vi "Tarea 8.vi"() -> ()   [LabVIEW 2020]
uses:
  <vilib>/addons/Control Design/_Model Construction/Model Creation.llb/Model Creation SubVI/cd_Create State Space Model.vi
  <vilib>/addons/Control Design/_Time Response Analysis/Time Response.llb/Time Response subVI/cd_Step Response (State-Space).vi
  <vilib>/addons/Control Design/_Dynamic Analysis/Dynamic Analysis.llb/Dynamic Analysis subVI/cd_Root Locus (State-Space).vi
  <vilib>/addons/Control Design/_Dynamic Analysis/Dynamic Analysis.llb/Dynamic Analysis subVI/cd_Poles (State-Space).vi
  <vilib>/addons/Control Design/_Utility/Model Viewer.llb/Model Viewer SubVI/cd_Draw Transfer Function Equation (SS).vi
  <vilib>/addons/Control Design/_Utility/Model Viewer.llb/Model Viewer SubVI/cd_Draw State-Space Equation (SS).vi
  <vilib>/imath/engines/lvmath/Plug In/Control Design/BuiltInFunctions/ackermann/NIMS_CD_ackermann(A,B,poles,STR).vi
  <vilib>/imath/engines/lvmath2/RunTimeEngine/ArithmeticOperatorToken/NIMS_ArithmeticOperator_multmx.vi
  <instcachedir>/0/NIMS_ArithmeticOperator_multmx_177F0753FB7A49B190E35F5DD0E80316.lvgen/NIMS_ArithmeticOperator_multmx_177F0753FB7A49B190E35F5DD0E80316_004.vi
  <vilib>/imath/engines/lvmath2/RunTimeEngine/ArithmeticOperatorToken/NIMS_ArithmeticOperator_minus.vi
  <instcachedir>/0/NIMS_ArithmeticOperator_minus_822089A08BE049DB927E6BEA78E100F1.lvgen/NIMS_ArithmeticOperator_minus_822089A08BE049DB927E6BEA78E100F1_002.vi
  <vilib>/imath/engines/lvmath2/RunTimeSupport/NIMS_Get Scalar_w Error.vi
  <instcachedir>/0/NIMS_Get Scalar_w Error_5A0E401CB6154DCF81784DB8E431B6E1.lvgen/NIMS_Get Scalar_w Error_5A0E401CB6154DCF81784DB8E431B6E1_003.vi
  <vilib>/imath/engines/lvmath2/RunTimeEngine/BuiltInFunctions/ss_to_tf/NIMS_ss_to_tf(4i).vi
  <vilib>/imath/engines/lvmath2/RunTimeEngine/ErrorHandling/NIMS_Create Error From Enums.vi
  <vilib>/imath/engines/lvmath/Plug In/Control Design/BuiltInFunctions/tf/NIMS_CD_tf(num,den,Ts).vi
  <vilib>/imath/engines/lvmath2/RunTimeEngine/NodeEndStatement/NIMS_NodeEndStatement_Output.vi
  <instcachedir>/0/NIMS_NodeEndStatement_Output_53EC0D466D134D7ABD903AC30B43404B.lvgen/NIMS_NodeEndStatement_Output_53EC0D466D134D7ABD903AC30B43404B_010.vi
  <instcachedir>/0/NIMS_NodeEndStatement_Output_53EC0D466D134D7ABD903AC30B43404B.lvgen/NIMS_NodeEndStatement_Output_53EC0D466D134D7ABD903AC30B43404B_005.vi
  <vilib>/imath/engines/lvmath2/RunTimeEngine/ErrorHandling/NIMS_Finalize Error.vi
  <vilib>/addons/Control Design/_Utility/Model Viewer.llb/Model Viewer SubVI/cd_Draw Transfer Function Equation (TF).vi
  <vilib>/addons/Control Design/_Utility/NI_CD_Model Viewer.lvlib
  <vilib>/addons/Control Design/_Model Construction/NI_LinSys_Model Creation.lvlib
  <vilib>/addons/Control Design/_State-Space Analysis/NI_CD_State-Space Analysis.lvlib
  <vilib>/addons/Control Design/_Dynamic Analysis/NI_CD_Dynamic Analysis.lvlib
  <vilib>/addons/Control Design/_Time Response Analysis/NI_CD_Time Response.lvlib
panel:
  out "TFO Equation":picture
  in  "Polos Observador":cdb[](array[numeric])=[-8.0+0.0i, -8.0+0.0i]
  out "ke":dbl[](array[numeric])
  out "Step Response Graph":cluster{"time":dbl[], dbl[]}[](graph)
  out "Root Locus Graph":cluster{dbl[], dbl[]}[](graph)
  out "Poles":cdb[](array[numeric]) format="%.3f"
  in  "Polos":cdb[](array[numeric])=[-2.0+3.4641i, -2.0-3.4641i, -10.0+0.0i]
  out "K":dbl[](array[numeric])
  out "Transfer Function Equation":picture
  out "Is Observable?":bool
  out "Observability  Matrix":dbl[][](array[numeric]) format="%#.2g"
  out "Is Controllable?":bool
  out "Controllability Matrix":dbl[][](array[numeric])=[[1.0, 0.0, 6.0], [0.0, 1.0, -1.0], [0.0, 0.0, 0.0]] format="%.2f"
  out "State Equation":picture
  in  "D":dbl[][](array[numeric])=[[1.0]]
  in  "C":dbl[][](array[numeric])=[[1.0, 1.0, 1.0]]
  in  "B":dbl[][](array[numeric])=[[1.0], [1.0], [1.0]]
  in  "A":dbl[][](array[numeric])=[[1.0, 1.0, 1.0], [1.0, 1.0, 1.0], [1.0, 1.0, 1.0]]
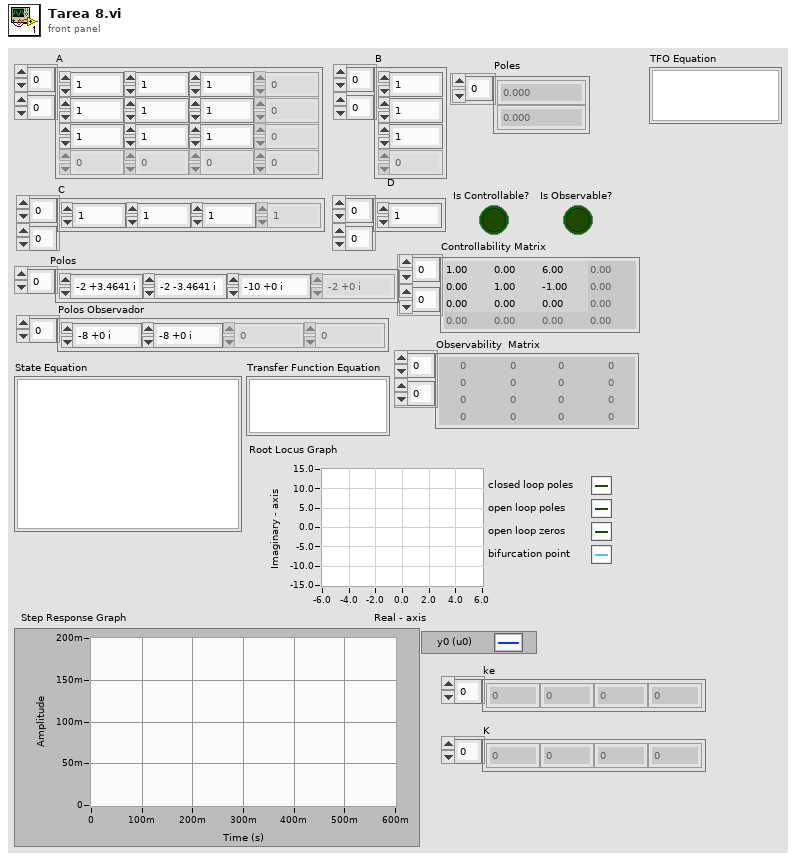
[diagram p1: front panel]
types:
  T1 = typedef "NI_LinSys_Model Typedefs.lvlib/CD State Space Model (MIMO).ctl" = cluster{"properties":T2, "A":dbl[][], "B":dbl[][], "C":dbl[][], "D":dbl[][], "StateNames":string[], "Transport Delay":dbl[][]}
  T2 = typedef "NI_LinSys_Model Typedefs.lvlib/CD General Elements.ctl" = cluster{"Model name":string, "Input names":string[], "Output names":string[], "Input Delays":dbl[], "Output Delays":dbl[], "Sampling Time":dbl, "Notes":string}
  T3 = typedef "NI_LinSys_Model Typedefs.lvlib/CD Transfer Function Model (MIMO).ctl" = cluster{"properties":T2, "transfer function(s)":T4[][]}
  T4 = typedef "NI_LinSys_Model Typedefs.lvlib/CD Transfer Function Model (SISO).ctl" = cluster{"Numerator":dbl[], "Denominator":dbl[], "delay":dbl}
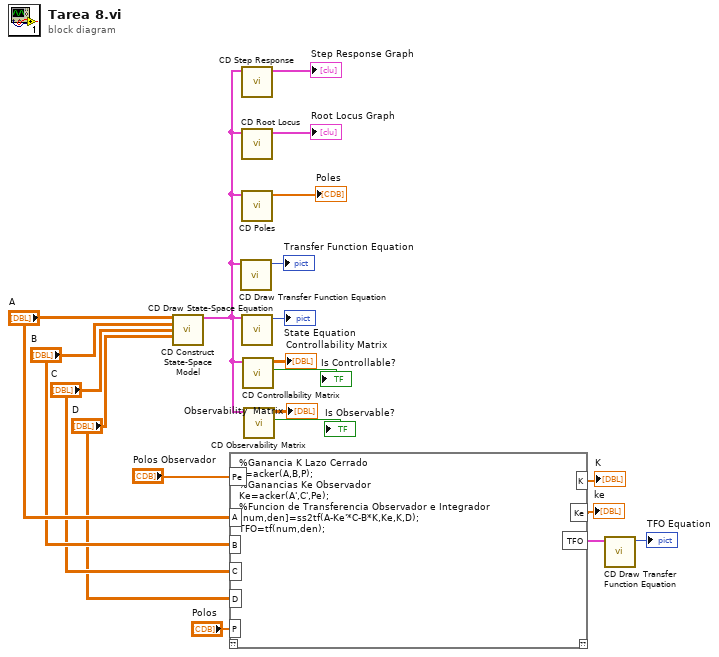
[diagram p0: block diagram]
diagram:
  n1 = call-poly <vilib>:"CD Construct State-Space Model.vi"("A"="A", "B"="B", "C"="C", "D"="D") -> ("State-Space Model"=w6:T1)  [unwired: 10 in, 1 out]
  n2 = mathscript code="%Ganancia K Lazo Cerrado\nK=acker(A,B,P);\n%Ganancias Ke Observador\nKe=acker(A',C',Pe);\n%Funcion de Transferencia Observador e Integrador\n[num,den]=ss2tf(A-Ke'*C-B*K,Ke,K,D);\nTFO=tf(num,den);"("A"="A", "B"="B", "C"="C", "D"="D", "P"="Polos", "Pe"="Polos Observador") -> ("K"=→"K":dbl[], "Ke"=→"ke":dbl[], "TFO"=w1:T3)  [unwired: 1 in, 1 out]
  n3 = call-poly <vilib>:"CD Draw Transfer Function Equation.vi"("State-Space Model"=w6) -> ("Equation"=→"Transfer Function Equation":picture)  [unwired: 8 in, 2 out]
  n4 = call-poly <vilib>:"CD Step Response.vi"("State-Space Model"=w6) -> ("Step Response Graph"=→"Step Response Graph":cluster{"time":dbl[], dbl[]}[])  [unwired: 7 in, 3 out]
  n5 = call-poly <vilib>:"CD Root Locus.vi"("State-Space Model"=w6) -> ("Root Locus Graph"=→"Root Locus Graph":cluster{dbl[], dbl[]}[])  [unwired: 7 in, 3 out]
  n6 = call-poly <vilib>:"CD Poles.vi"("State-Space Model"=w6) -> ("Poles"=→"Poles":cdb[])  [unwired: 9 in, 1 out]
  n7 = call-poly <vilib>:"CD Draw State-Space Equation.vi"("State-Space Model"=w6) -> ("Equation"=→"State Equation":picture)  [unwired: 8 in, 2 out]
  n8 = call <vilib>:"CD Controllability Matrix.vi"("State-Space Model"=w6) -> ("Is Controllable?"=→"Is Controllable?":bool, "Controllability Matrix"=→"Controllability Matrix":dbl[][])  [unwired: 7 in, 2 out]
  n9 = call <vilib>:"CD Observability Matrix.vi"("State-Space Model"=w6) -> ("Is Observable?"=→"Is Observable?":bool, "Observability  Matrix"=→"Observability  Matrix":dbl[][])  [unwired: 7 in, 2 out]
  n10 = call-poly <vilib>:"CD Draw Transfer Function Equation.vi"("Transfer Function Model"=w1) -> ("Equation"=→"TFO Equation":picture)  [unwired: 8 in, 2 out]
